vi "Set DAQ timing to Sample Complete.vi"(8 "error in (no error)":errorcluster, 11 "Target":refnum<k24>) -> (0 "error out":errorcluster, 3 "Target out":refnum<k24>)   [LabVIEW 2020]
uses:
  NationalInstruments.VeriStand.SystemDefinitionAPI
  NationalInstruments.VeriStand.SystemStorage
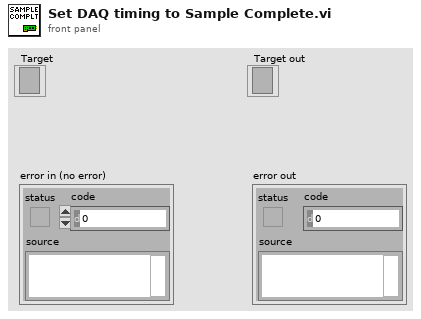
[diagram p1: front panel]
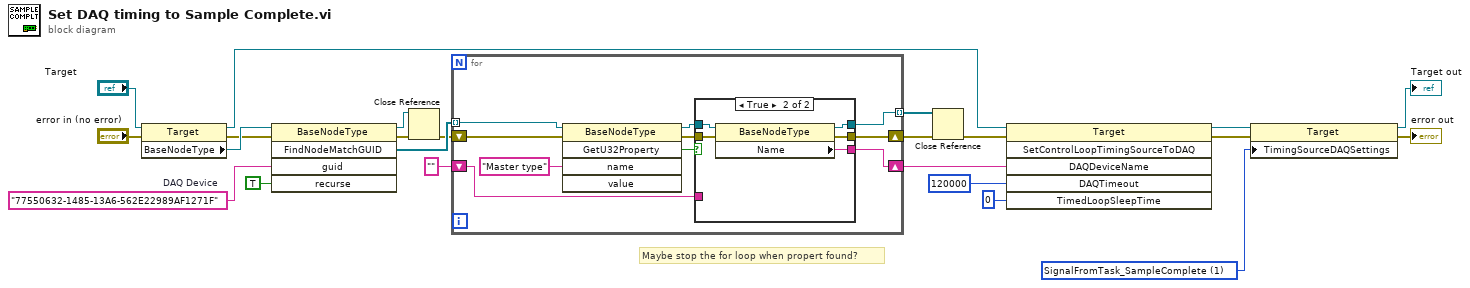
[diagram p0: block diagram]
diagram:
  w13 = "77550632-1485-13A6-562E22989AF1271F"  # DAQ Device
  w19 = 1 items=["ControlLoopFromTask", "SignalFromTask_SampleComplete"] ("TimingSourceDAQSettings")
  # "Maybe stop the for loop when propert found?"
  n1 = property class="Target"(reference="Target", error in="error in (no error)") -> (reference out=w11:refnum<k24>, error out=w7:errorcluster, "BaseNodeType"=w14:refnum<k24>)
  n2 = invoke class="BaseNodeType" method="FindNodeMatchGUID"(reference=w14, error in=w7, "guid"=w13, "recurse"=TRUE) -> (reference out=w4:refnum<k24>, error out=w6:errorcluster, "FindNodeMatchGUID"=w10:refnum<k24>[])  [unwired: 1 in, 2 out]
  n3 = Close Reference(reference=w4, error in (no error)=w6) -> (error out=w5:errorcluster)
  n4 = for {
    tunnel: w10 -> [w33] mode=indexing
    shift-right: [w29] -> w8
    shift-left: "" ("name") -> [w28]
    shift-right: [w25] -> w3
    shift-left: w5 -> [w27]
    tunnel: [w24] -> w1 mode=indexing
    n5 = invoke class="BaseNodeType" method="GetU32Property"(reference=w33, error in=w27, "name"="Master type") -> (reference out=w30:refnum<k24>, error out=w26:errorcluster, "GetU32Property"=w31:bool)  [unwired: 2 in, 2 out]
    n6 = case shown="True" w31 {
      tunnel: w30 -> [w34 w41]
      tunnel: [w36 w40] -> w29
      tunnel: w28 -> [w36 _]
      tunnel: w26 -> [w35 w39]
      tunnel: [w35 w38] -> w25
      tunnel: [w34 w37] -> w24
      frame False {
      }
      frame True {
        n7 = property class="BaseNodeType"(reference=w41, error in=w39) -> (reference out=w37:refnum<k24>, error out=w38:errorcluster, "Name"=w40:string)
      }
    }
  }
  n8 = Close Reference(reference=w1, error in (no error)=w3) -> (error out=w2:errorcluster)
  n9 = invoke class="Target" method="SetControlLoopTimingSourceToDAQ"(reference=w11, error in=w2, "DAQDeviceName"=w8, "DAQTimeout"=u32 120000, "TimedLoopSleepTime"=u32 0) -> (reference out=w16:refnum<k24>, error out=w15:errorcluster)  [unwired: 1 in, 4 out]
  n10 = property class="Target"(reference=w16, error in=w15, "TimingSourceDAQSettings"=w19) -> (reference out=→"Target out":refnum<k24>, error out=→"error out":errorcluster)
